vi "ActionVIOnDelete_Controller.vi"(6 "All deleted Refs":T1[](array[typedef]) format="%.0x", 8 "error in (no error)":errorcluster, 11 "Item Ref in":T1 format="%.0x") -> (0 "error out":errorcluster, 3 "Item Ref out":T1 format="%.0x")   [LabVIEW 2019, in "Control Addon System Explorer.lvlib"]
uses:
  Control Addon System Explorer.lvlib
  <vilib>/NI VeriStand/Custom Device API/Custom Device Item Ref.ctl
  Addon Shared/Control Addon Shared.lvlib
  <vilib>/NI VeriStand/Custom Device API/Custom Device API.lvlib
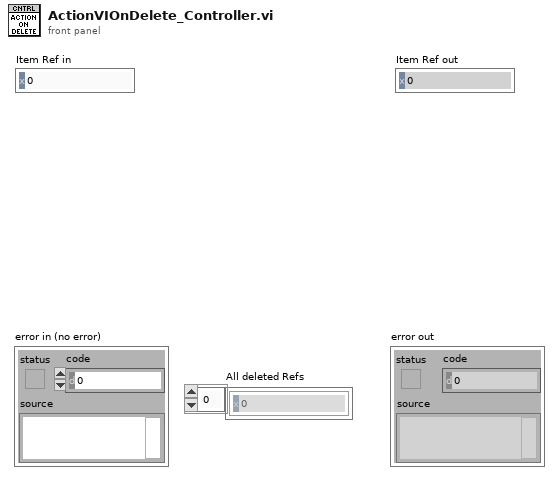
[diagram p1: front panel]
types:
  T1 = typedef "Custom Device API.lvlib/Custom Device Item Ref.ctl" = u64
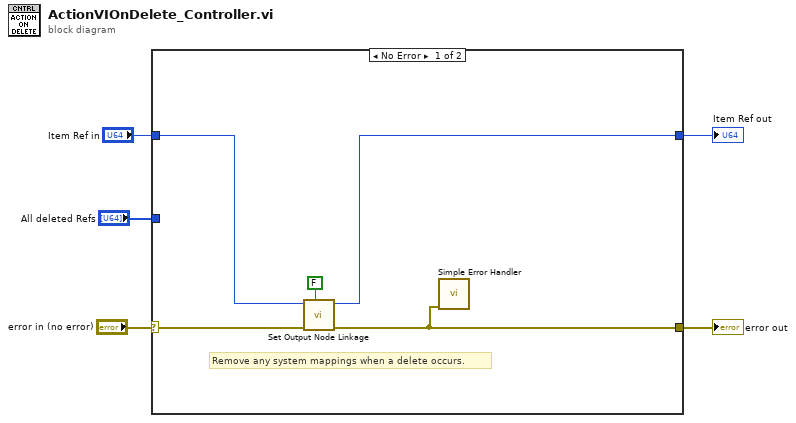
[diagram p0: block diagram]
diagram:
  n1 = case shown="No Error" "error in (no error)" {
    selector: "error in (no error)" -> [w6 w12]
    tunnel: [w8 w12] -> w4
    tunnel: "Item Ref in" -> [w7 w11]
    tunnel: [w9 w11] -> w2
    tunnel: "All deleted Refs" -> [_ _]
    frame No Error {
      # "Remove any system mappings when a delete occurs."
      n2 = call "Set Output Node Linkage.vi"("Add?"=FALSE ("Add? (T)"), "error in"=w6, "Section Ref in"=w7) -> ("error out"=w8:errorcluster, "Item Ref out"=w9:T1)  [unwired: 7 in]
      n3 = call <vilib>:"Simple Error Handler.vi"("error in (no error)"=w8) -> ()  [unwired: 4 in, 5 out]
    }
    frame Error {
    }
  }
  "error out" <- w4
  "Item Ref out" <- w2
